vi "set force wire mode.vi"(8 "error in":errorcluster, 10 "force wire mode":bool, 11 "Modbus Slave configuration in":refnum<class "Modbus Module configuration.lvclass">) -> (0 "error out":errorcluster, 3 "Modbus Slave configuration out":refnum<class "Modbus Module configuration.lvclass">)   [LabVIEW 2015, in "Modbus Module configuration.lvclass"]
uses:
  Modbus Module configuration.lvclass
  Modbus Module configuration.lvclass/Modbus Module configuration.ctl
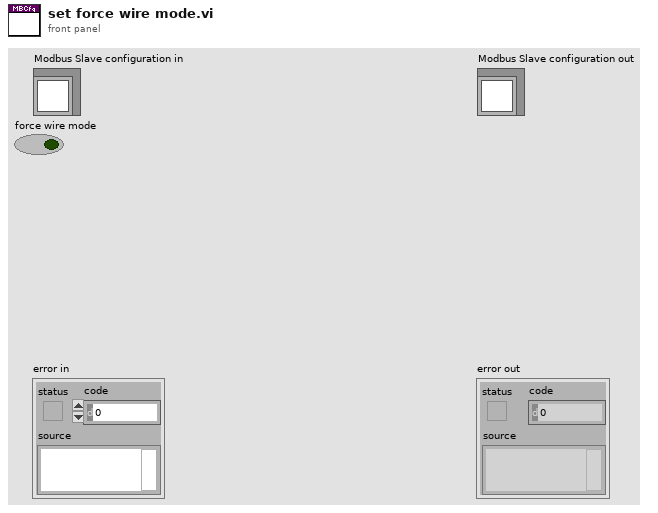
[diagram p1: front panel]
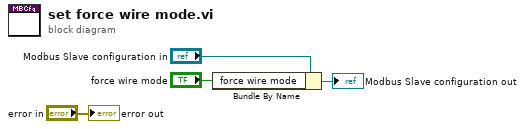
[diagram p0: block diagram]
diagram:
  n1 = Bundle By Name(cluster="Modbus Slave configuration in", "force wire mode"="force wire mode") -> (→"Modbus Slave configuration out":refnum<class "Modbus Module configuration.lvclass">)
  "error out" <- "error in"
